vi "SQL Statement probe.vi"(11 "SQL Statement in":refnum<class "SQL Statement.lvclass">) -> (2 "Value String":string, 3 "Boolean":bool)   [LabVIEW 2013, in "SQLiteSupport.lvlib" / "SQL Statement.lvclass"]
uses:
  SQL Statement/SQL Statement.lvclass
panel:
  out "Prepared SQL Statement":string
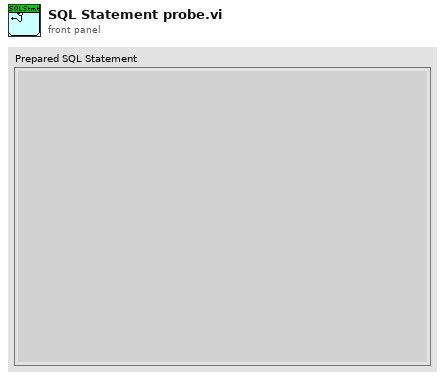
[diagram p1: front panel]
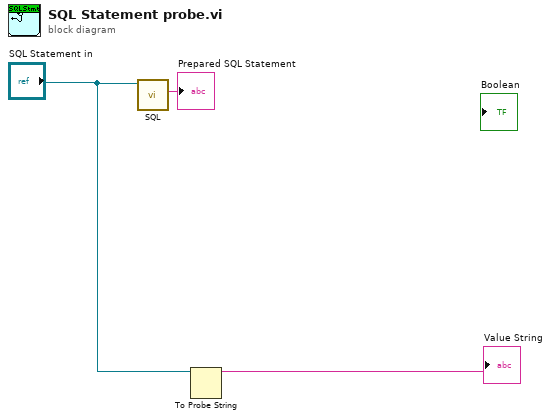
[diagram p0: block diagram]
diagram:
  n1 = call "SQL.vi"("SQL Statement in"="SQL Statement in") -> ("SQL"=→"Prepared SQL Statement":string)  [unwired: 8 in, 2 out]
  n2 = To Probe String(7:"SQL Statement in") -> (3:→"Value String":string)  [unwired: 2 in, 1 out]
